vi "Shut Down Device.vi"(8 "error in (no error)":errorcluster, 11 "cetoni in":refnum<class "PHD Ultra.lvclass">) -> (0 "error out":errorcluster, 3 "cetoni out":refnum<class "PHD Ultra.lvclass">)   [LabVIEW 2018, in "PHD Ultra.lvlib" / "PHD Ultra.lvclass"]
uses:
  PHD Ultra.lvclass
  PHD Ultra.lvclass/PHD Ultra.ctl
  Device/Device.lvclass
  <userlib>/QmixLib/QmixLib.lvlib
  Program Files/cetoni/QmixSDK/lib/labview/labbCAN_Pump_API/labbCAN_Pump_API.lvlib
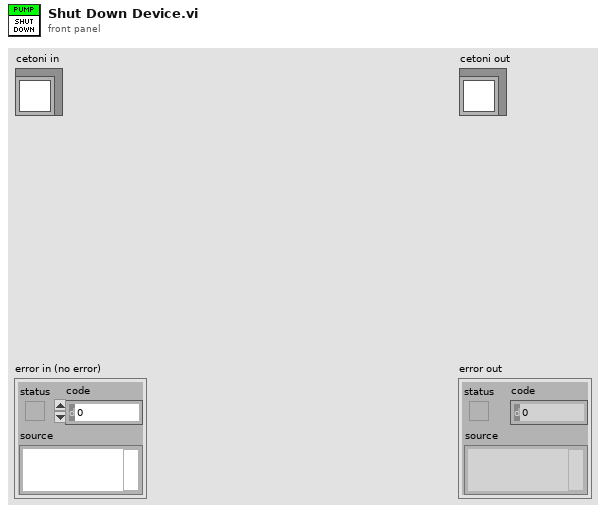
[diagram p1: front panel]
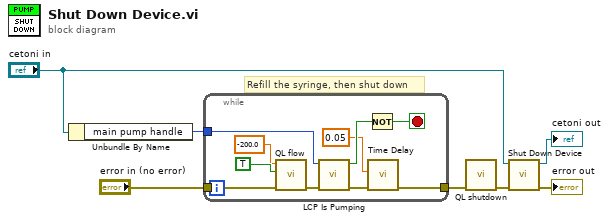
[diagram p0: block diagram]
diagram:
  # "Refill the syringe, then shut down"
  n1 = Unbundle By Name("cetoni in") -> ("main pump handle"=w3:i64)
  n2 = while {
    tunnel: w3 -> [w15]
    tunnel: "error in (no error)" -> [w12]
    tunnel: [w10] -> w1
    stop <- w17 stop-if-true
    n3 = call <userlib>:"QL flow.vi"("error in (no error)"=w12, "auto_switch_valve"=TRUE, "flow_rate_uL_s"=-200.0) -> ("error out"=w14:errorcluster)  [unwired: 8 in]
    n4 = call "LCP Is Pumping.vi"("error in (no error)"=w14, "Pump Handle"=w15) -> ("error out"=w11:errorcluster, "Is pumping"=w16:bool)  [unwired: 8 in]
    n5 = Not(x=w16) -> (.not. x?=w17:bool)
    n6 = call "Time Delay"("error in (no error)"=w11, "Delay Time (s)"=0.05) -> ("error out"=w10:errorcluster)  [unwired: 9 in]
  }
  n7 = call <userlib>:"QL shutdown.vi"("error in (no error)"=w1) -> ("error out"=w5:errorcluster)  [unwired: 10 in]
  n8 = call-parent "Shut Down Device.vi"("error in (no error)"=w5, "Device in"="cetoni in") -> ("error out"=→"error out":errorcluster, "Device out"=→"cetoni out":refnum<class "PHD Ultra.lvclass">)  [unwired: 8 in]
